vi "Delete Previous Item Descendants.vi"(8 "error in (no error)":errorcluster, 10 "Edit Tree Items:Add Item to End":string, 11 "TreeControl in":refnum<vi>) -> (0 "error out":errorcluster, 3 "TreeControl out":refnum<vi>)   [LabVIEW 2020, in "Peek Window.lvlib"]
uses:
  Peek Window.lvlib
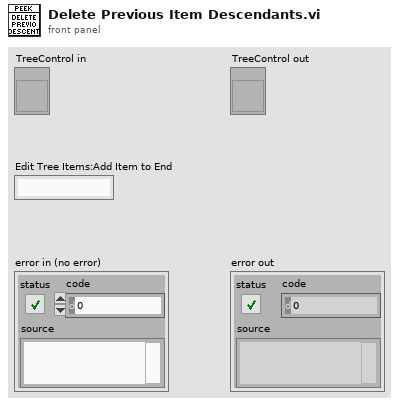
[diagram p1: front panel]
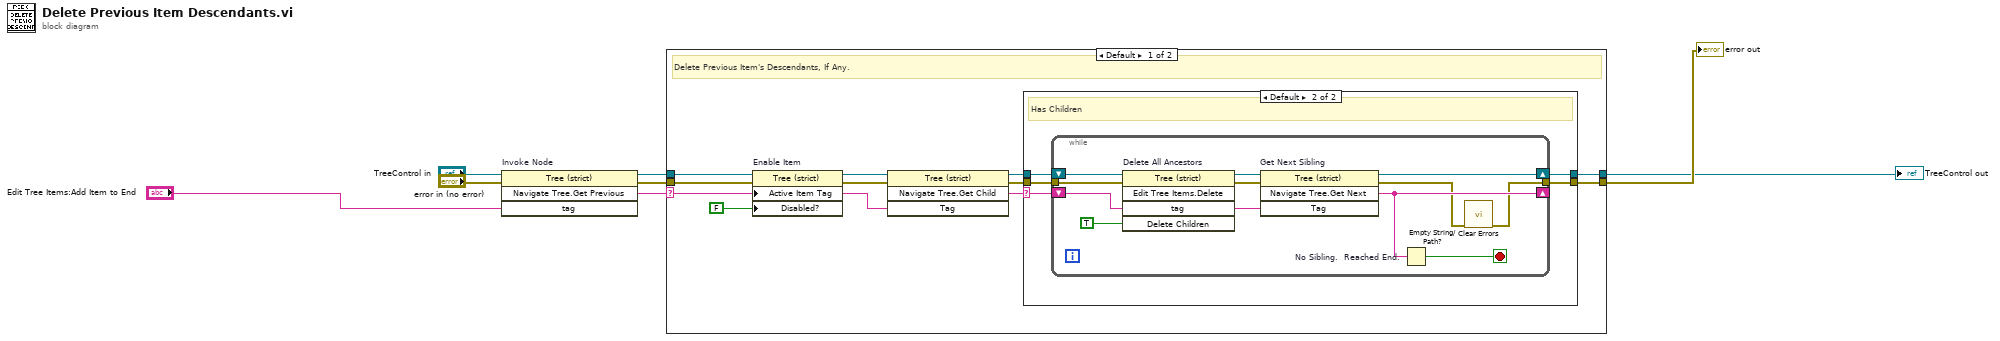
[diagram p0: block diagram]
diagram:
  n1 = invoke on="Invoke Node" class="Tree (strict)" method="Navigate Tree.Get Previous"(reference="TreeControl in", error in="error in (no error)", "tag"="Edit Tree Items:Add Item to End") -> (reference out=w6:refnum<vi>, error out=w5:errorcluster, "Navigate Tree:Get Previous"=w4:string)  [unwired: 1 in, 1 out]
  n2 = case shown="Default" w4 {
    selector: w4 -> [w10 _]
    tunnel: w5 -> [w15 w39]
    tunnel: [w16 w39] -> w8
    tunnel: w6 -> [w12 w38]
    tunnel: [w14 w38] -> w7
    frame Default {
      # "Delete Previous Item's Descendants, If Any."
      n3 = property on="Enable Item" class="Tree (strict)"(reference=w12, error in=w15, "Active Item Tag"=w10, "Disabled?"=FALSE) -> (reference out=w11:refnum<vi>, error out=w13:errorcluster)
      n4 = invoke class="Tree (strict)" method="Navigate Tree.Get Child"(reference=w11, error in=w13, "Tag"=w10) -> (reference out=w18:refnum<vi>, error out=w19:errorcluster, "Navigate Tree:Get Child"=w17:string)  [unwired: 1 in, 1 out]
      n5 = case shown="Default" w17 {
        selector: w17 -> [_ w24]
        tunnel: w19 -> [w21 w26]
        tunnel: w18 -> [w20 w25]
        tunnel: [w21 w23] -> w16
        tunnel: [w20 w22] -> w14
        frame "" {
          # "No Children"
        }
        frame Default {
          # "Has Children"
          n6 = while {
            tunnel: w26 -> [w34]
            shift-right: [w30] -> w22
            shift-left: w25 -> [w35]
            tunnel: [w27] -> w23
            shift-right: [w29] -> _
            shift-left: w24 -> [w33]
            stop <- w36 stop-if-true
            n7 = invoke on="Delete All Ancestors" class="Tree (strict)" method="Edit Tree Items.Delete"(reference=w35, error in=w34, "tag"=w33, "Delete Children"=TRUE) -> (reference out=w31:refnum<vi>, error out=w32:errorcluster)  [unwired: 1 in, 3 out]
            n8 = invoke on="Get Next Sibling" class="Tree (strict)" method="Navigate Tree.Get Next"(reference=w31, error in=w32, "Tag"=w33) -> (reference out=w30:refnum<vi>, error out=w28:errorcluster, "Navigate Tree:Get Next Item"=w29:string)  [unwired: 1 in, 1 out]
            n9 = Empty String/Path? "No Sibling.  Reached End."(string/path=w29) -> (empty?=w36:bool)
            n10 = call <vilib>:"Clear Errors.vi"("error in (no error)"=w28) -> ("error out"=w27:errorcluster)  [unwired: 5 in, 1 out]
          }
        }
      }
    }
    frame "" {
      # "No Previous Item."
    }
  }
  "error out" <- w8
  "TreeControl out" <- w7
